vi "Event Handle Loop_Draw.vi"(8 "error in (no error)":errorcluster, 11 "QMenu Class in":refnum<class "QMenu Class.lvclass">) -> (0 "error out":errorcluster, 3 "QMenu Class out":refnum<class "QMenu Class.lvclass">)   [LabVIEW 2020, in "QTab.lvlib" / "QMenu Class.lvclass"]
uses:
  QMenu Class.lvclass
  QMenu Class.lvclass/QMenu Class.ctl
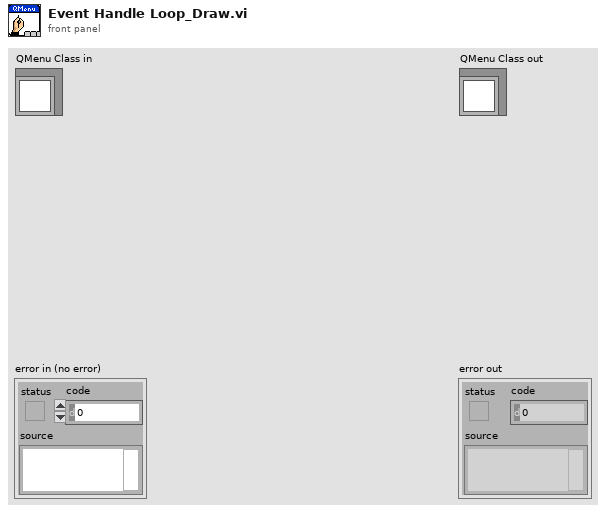
[diagram p1: front panel]
types:
  T1 = typedef "QTab.lvlib/QMenu Class.lvclass/Button Attribute.ctl" = cluster{"Label":string, "Button Text":string, "Closable":bool, "Draggable":bool}
  T2 = typedef "imagedata.ctl" = cluster{"image type":i32, "image depth":i32, "image":u8[], "mask":u8[], "colors":u32[], "Rectangle":cluster{"left":i16, "top":i16, "right":i16, "bottom":i16}}
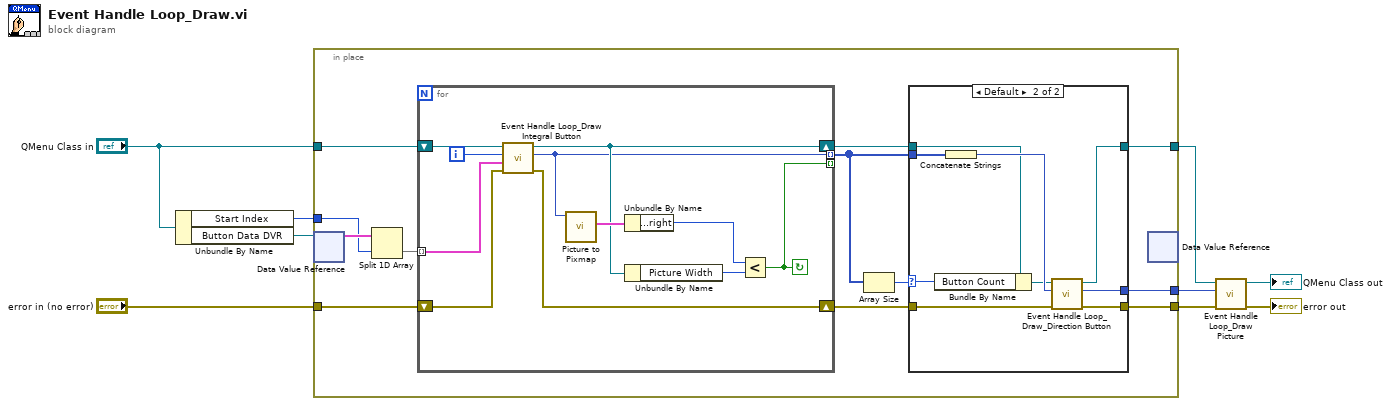
[diagram p0: block diagram]
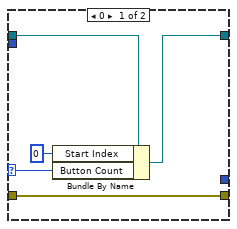
[diagram p2: hidden frame]
diagram:
  n1 = Unbundle By Name("QMenu Class in") -> ("Start Index"=w8:i32, "Button Data DVR"=w9:refnum<data-value>)
  n2 = in-place {
    in-place-border: "QMenu Class in" -> [w21]
    in-place-border: [w15] -> w3
    in-place-border: "error in (no error)" -> [w20]
    in-place-border: [w14] -> w5
    in-place-border: w8 -> [w17]
    in-place-border: [w13] -> w4
    n3 = in-place-dvr #1(w9) -> (w18:T1[])  [unwired: 1 out]
    n4 = Split 1D Array(array=w18, index=w17) -> (second subarray=w19:T1[])  [unwired: 1 out]
    n5 = for {
      tunnel: w19 -> [w44] mode=indexing
      shift-right: [w40] -> w11
      shift-left: w21 -> [w46]
      shift-right: [w41] -> w16
      shift-left: w20 -> [w45]
      tunnel: [w36] -> w12 mode=indexing if=w37
      tunnel: [w37] -> _ mode=indexing
      i -> [w38]
      stop <- w37 continue-if-true
      n6 = call "Event Handle Loop_Draw Integral Button.vi"("error in (no error)"=w45, "Button Attribute"=w44, "Index"=w38, "QMenu Class in"=w46) -> ("error out"=w41:errorcluster, "Picture"=w36:picture, "QMenu Class out"=w40:refnum<class "QMenu Class.lvclass">)  [unwired: 5 in]
      n7 = call <vilib>:"Picture to Pixmap.vi"("picture"=w36) -> ("image data"=w43:T2)  [unwired: 9 in, 1 out]
      n8 = Unbundle By Name(w43) -> ("Rectangle.right"=w39:i16)
      n9 = Unbundle By Name(w40) -> ("Picture Width"=w42:i16)
      n10 = Less?(x=w39, y=w42) -> (x < y?=w37:bool)
    }
    n11 = Array Size(array=w12) -> (size(s)=w10:i32)
    n12 = case shown="Default" w10 {
      selector: w10 -> [w24 w29]
      tunnel: w16 -> [w26 w35]
      tunnel: w11 -> [w25 w28]
      tunnel: [w23 w34] -> w15
      tunnel: [w26 w33] -> w14
      tunnel: [_ w32] -> w13
      tunnel: w12 -> [_ w31]
      frame 0 {
        n13 = Bundle By Name(cluster=w25, "Start Index"=0 ("Buffer Data.Start Index"), "Button Count"=w24) -> (w23:refnum<class "QMenu Class.lvclass">)
      }
      frame Default {
        n14 = Bundle By Name(cluster=w28, "Button Count"=w29) -> (w27:refnum<class "QMenu Class.lvclass">)
        n15 = Concatenate Strings(w31) -> (w30:picture)
        n16 = call "Event Handle Loop_Draw_Direction Button.vi"("error in (no error)"=w35, "Picture In"=w30, "QMenu Class in"=w27) -> ("error out"=w33:errorcluster, "Picture Out"=w32:picture, "QMenu Class out"=w34:refnum<class "QMenu Class.lvclass">)  [unwired: 6 in]
      }
    }
    n17 = in-place-dvr #1() -> ()  [unwired: 1 in, 2 out]
  }
  n18 = call "Event Handle Loop_Draw Picture.vi"("error in (no error)"=w5, "Picture"=w4, "QMenu Class in"=w3) -> ("error out"=→"error out":errorcluster, "QMenu Class out"=→"QMenu Class out":refnum<class "QMenu Class.lvclass">)  [unwired: 7 in]
